vi "Open VI by Test Name.vi"(8 "error in (no error)":errorcluster, 11 "Tag":string) -> (0 "error in (no error) 2":errorcluster)   [LabVIEW 2020, in "Execution UI.lvclass"]
uses:
  Execution UI.lvclass
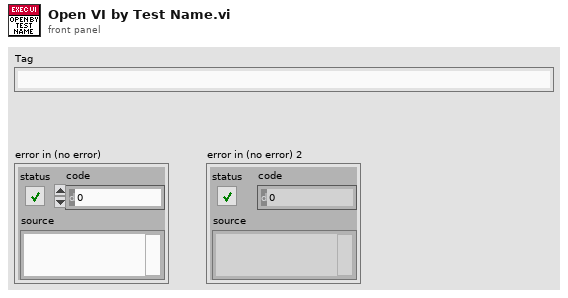
[diagram p1: front panel]
types:
  T1 = enum32{"Invalid", "Standard", "Closed", "Hidden", "Minimized", "Maximized"}
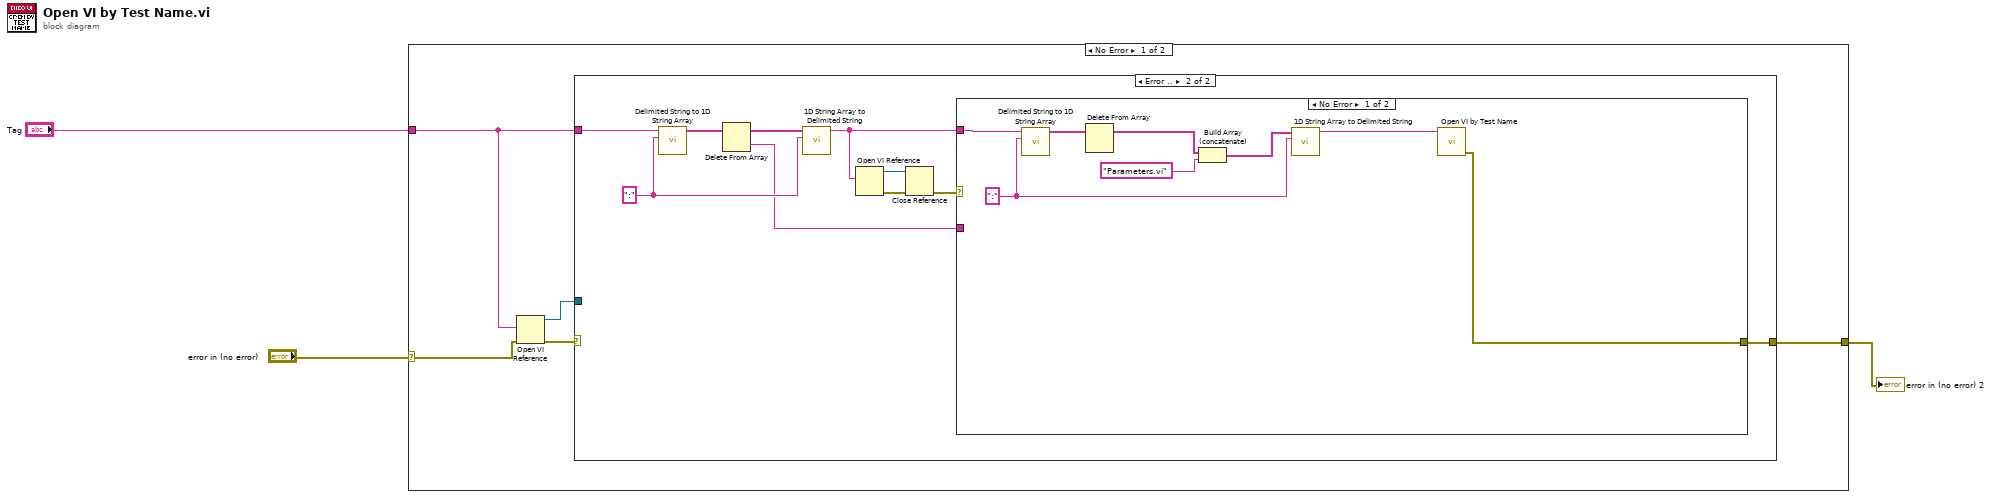
[diagram p0: block diagram]
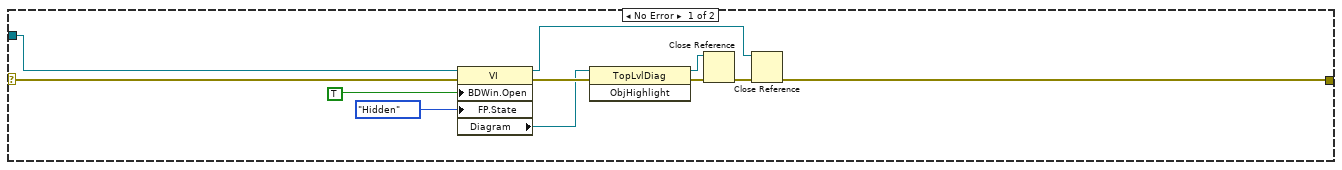
[diagram p2: hidden frame]
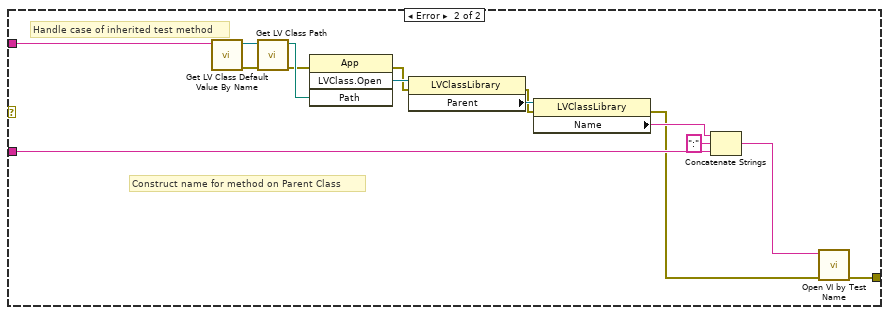
[diagram p3: hidden frame]
diagram:
  n1 = case shown="No Error" "error in (no error)" {
    selector: "error in (no error)" -> [w5 w53]
    tunnel: "Tag" -> [w6 _]
    tunnel: [w4 w53] -> w1
    frame No Error {
      n2 = Open VI Reference(vi path=w6, error in (no error)=w5) -> (vi reference=w8:refnum<vi>, error out=w7:errorcluster)  [unwired: 4 in]
      n3 = case shown="Error .." w7 {
        selector: w7 -> [w14 _]
        tunnel: w8 -> [w16 _]
        tunnel: w6 -> [_ w26]
        tunnel: [w19 w24] -> w4
        frame No Error {
          n4 = property class="VI"(reference=w16, error in=w14, "BDWin.Open"=TRUE ("Block Diagram Window:Open"), "FP.State"=T1."Hidden" ("Front Panel Window:State")) -> (reference out=w17:refnum<vi>, error out=w15:errorcluster, "Diagram"=w11:refnum<vi>)
          n5 = invoke class="TopLvlDiag" method="ObjHighlight"(reference=w11, error in=w15) -> (reference out=w9:refnum<vi>, error out=w12:errorcluster)  [unwired: 1 in, 1 out]
          n6 = Close Reference(reference=w9, error in (no error)=w12) -> (error out=w10:errorcluster)
          n7 = Close Reference(reference=w17, error in (no error)=w10) -> (error out=w19:errorcluster)
        }
        frame Error {
          w27 = ":" ("delimiter")
          n8 = call <vilib>:"Delimited String to 1D String Array.vi"("delimiter"=w27, "delimited string"=w26) -> ("string array"=w28:string[])  [unwired: 9 in]
          n9 = Delete From Array(array=w28) -> (deleted portion=w25:string, array with subset deleted=w29:string[])  [unwired: 2 in]
          n10 = call <vilib>:"1D String Array to Delimited String.vi"("delimiter"=w27, "string array"=w29) -> ("delimited string"=w23:string)  [unwired: 9 in]
          n11 = Open VI Reference(vi path=w23) -> (vi reference=w20:refnum<vi>, error out=w22:errorcluster)  [unwired: 5 in]
          n12 = Close Reference(reference=w20, error in (no error)=w22) -> (error out=w21:errorcluster)
          n13 = case shown="No Error" w21 {
            tunnel: w25 -> [_ w45]
            tunnel: [w30 w43] -> w24
            tunnel: w23 -> [w35 w38]
            frame No Error {
              w36 = ":" ("delimiter")
              n14 = call <vilib>:"Delimited String to 1D String Array.vi"("delimiter"=w36, "delimited string"=w35) -> ("string array"=w37:string[])  [unwired: 9 in]
              n15 = Delete From Array(array=w37) -> (array with subset deleted=w34:string[])  [unwired: 2 in, 1 out]
              n16 = Build Array (concatenate)(w34, "Parameters.vi" ("string")) -> (w32:string[])
              n17 = call <vilib>:"1D String Array to Delimited String.vi"("delimiter"=w36, "string array"=w32) -> ("delimited string"=w31:string)  [unwired: 9 in]
              n18 = call "Open VI by Test Name.vi"("Tag"=w31) -> ("error in (no error) 2"=w30:errorcluster)  [unwired: 10 in]
            }
            frame Error {
              # "Handle case of inherited test method"
              # "Construct name for method on Parent Class"
              n19 = call <vilib>:"Get LV Class Default Value By Name.vi"("class name"=w38) -> ("error out"=w52:errorcluster, "object"=w51:refnum<class>)  [unwired: 9 in]
              n20 = call <vilib>:"Get LV Class Path.vi"("error in (no error)"=w52, "object"=w51) -> ("error out"=w49:errorcluster, "class path"=w50:path)  [unwired: 8 in]
              n21 = invoke class="App" method="LVClass.Open"(error in=w49, "Path"=w50) -> (error out=w40:errorcluster, "LVClass.Open"=w48:refnum<vi>)  [unwired: 2 in, 2 out]
              n22 = property class="LVClassLibrary"(reference=w48, error in=w40) -> (error out=w41:errorcluster, "Parent"=w47:refnum<vi>)  [unwired: 1 out]
              n23 = property class="LVClassLibrary"(reference=w47, error in=w41) -> (error out=w42:errorcluster, "Name"=w46:string)  [unwired: 1 out]
              n24 = Concatenate Strings(w46, ":" ("string"), w45) -> (w44:string)
              n25 = call "Open VI by Test Name.vi"("error in (no error)"=w42, "Tag"=w44) -> ("error in (no error) 2"=w43:errorcluster)  [unwired: 9 in]
            }
          }
        }
      }
    }
    frame Error {
    }
  }
  "error in (no error) 2" <- w1
